vi "SimpleSSHTest.vi"() -> ()   [LabVIEW 2020]
panel:
  out "concatenated string":string
  in  "stop":bool
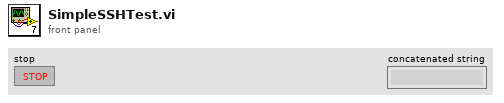
[diagram p1: front panel]
types:
  T1 = cluster{"IP Address":string, "Username":string, "password":string}
  T2 = typedef "PythonCtrl.ctl" = cluster{"session":refnum<k35>, "PyPath":path, "Processor":enum16{"SPIKE", "Pi", "Pi_ssh"}}
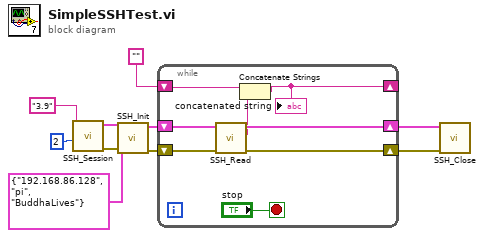
[diagram p0: block diagram]
diagram:
  n1 = call "SSH_Session.vi"("Processor"=2, "Python version"="3.9") -> ("error out"=w9:errorcluster, "Python"=w8:T2)  [unwired: 8 in]
  n2 = call "SSH_Init.vi"("error in (no error)"=w9, "Raspberry Pi"=T1 {"IP Address"="192.168.86.128", "Username"="pi", "password"="BuddhaLives"}, "Python in"=w8) -> ("error out"=w6:errorcluster, "Python out"=w5:T2)  [unwired: 6 in, 1 out]
  n3 = while {
    shift-right: [w16] -> w4
    shift-left: w6 -> [w18]
    shift-right: [w15] -> w3
    shift-left: w5 -> [w17]
    shift-right: [w11] -> _
    shift-left: "" ("Reply") -> [w12]
    stop <- "stop" stop-if-true
    n4 = call "SSH_Read.vi"("error in (no error)"=w18, "Python"=w17) -> ("error out"=w16:errorcluster, "Reply"=w13:string, "Python"=w15:T2)  [unwired: 7 in]
    n5 = Concatenate Strings(w12, w13) -> (w11:string)
    "concatenated string" <- w11
  }
  n6 = call "SSH_Close.vi"("error in (no error)"=w4, "Python"=w3) -> ()  [unwired: 9 in, 1 out]
